vi "to string array.vi"(8 "error in (no error)":errorcluster, 11 "module configuration in":refnum<class "tag bus configurable plugin module configuration.lvclass">) -> (0 "error out":errorcluster, 1 "Array":string[][](array[string]), 2 "version":string, 3 "module configuration out":refnum<class "tag bus configurable plugin module configuration.lvclass">)   [LabVIEW 2014, in "tag bus configurable plugin module configuration.lvclass"]
uses:
  tag bus configurable plugin module configuration.lvclass
  tag bus configurable plugin module configuration.lvclass/tag bus configurable plugin module configuration.ctl
  <vilib>/NI/Tag Bus/tag/tag descriptor.lvclass/tag descriptor.ctl
  <vilib>/NI/Tag Bus Module Framework/channel/TBM channel.lvclass/TBM channel.ctl
  Read Lines.vi
  <vilib>/NI/Tag Bus Module Framework/channel/TBM channel.lvclass
  <vilib>/NI/Tag Bus/tag/tag descriptor.lvclass
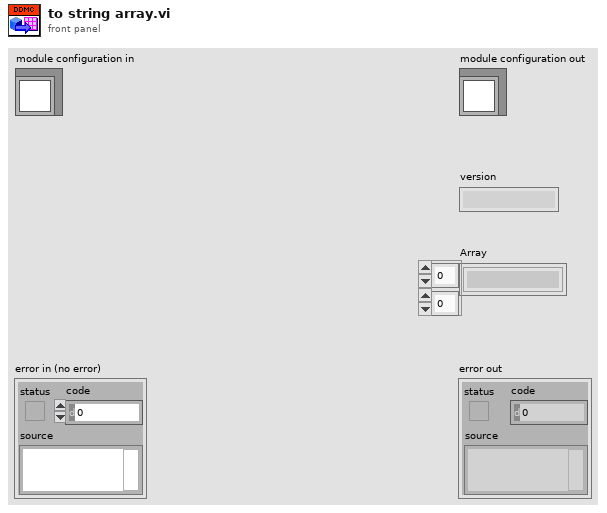
[diagram p1: front panel]
types:
  T1 = typedef "tag bus configurable plugin module configuration.lvclass/Line.ctl" = cluster{"channel":refnum<class "TBM channel.lvclass">}
  T2 = typedef "TBM channel.lvclass/channel classification.ctl" = enum16{"input data", "output data", "processing parameter", "processing result"}
  T3 = typedef "tag bus.lvlib/tag descriptor.lvclass/Data Type.ctl" = enum16{"Double", "Single", "I64", "I32", "I16", "I8", "U64", "U32", "U16", "U8", "Boolean", "String", "Array of Double", "Array of Single", "Array of I64", "Array of I32", "Array of I16", "Array of I8", "Array of U64", "Array of U32", "Array of U16", "Array of U8", "Array of Boolean", "Array of String"}
  T4 = typedef "tag bus configurable plugin module configuration.lvclass/permissions.ctl" = enum32{"Read from HW", "Write to HW"}
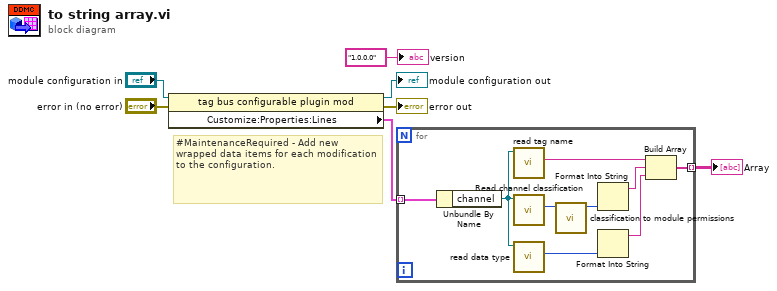
[diagram p0: block diagram]
diagram:
  # "#MaintenanceRequired - Add new wrapped data items for each modification to the configuration."
  n1 = property class="tag bus configurable plugin mod"(reference="module configuration in", error in="error in (no error)") -> (reference out=→"module configuration out":refnum<class "tag bus configurable plugin module configuration.lvclass">, error out=→"error out":errorcluster, "Customize:Properties:Lines"=w4:T1[])
  n2 = for {
    tunnel: w4 -> [w16] mode=indexing
    tunnel: [w8] -> w1 mode=indexing
    n3 = Unbundle By Name(w16) -> ("channel"=w11:refnum<class "TBM channel.lvclass">)
    n4 = call <vilib>:"read tag name.vi"("system tag in"=w11) -> ("name"=w15:string)  [unwired: 8 in, 2 out]
    n5 = call <vilib>:"Read channel classification.vi"("channel in"=w11) -> ("channel classification"=w14:T2)  [unwired: 8 in, 2 out]
    n6 = call <vilib>:"read data type.vi"("system tag in"=w11) -> ("data type"=w10:T3)  [unwired: 8 in, 2 out]
    n7 = call "classification to module permissions.vi"("channel classification"=w14) -> ("permissions"=w13:T4)  [unwired: 10 in]
    n8 = Format Into String(w13) -> (resulting string=w12:string)  [unwired: 3 in, 1 out]
    n9 = Format Into String(w10) -> (resulting string=w9:string)  [unwired: 3 in, 1 out]
    n10 = Build Array(w15, w12, w9) -> (w8:string[])
  }
  "Array" <- w1
  "version" <- "1.0.0.0" ("version")
